vi "Make Project Title string.vi"(6 "Version":string, 8 "Simulate?":bool, 9 "Debug?":bool, 10 "Project Name":string) -> (3 "Title Bar":string)   [LabVIEW 2013, in "Strings Lib.lvlib"]
doc: "Formats the title bar string."
uses:
  Strings Lib.lvlib
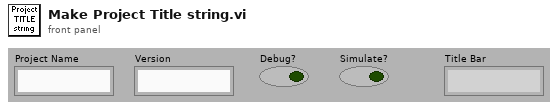
[diagram p1: front panel]
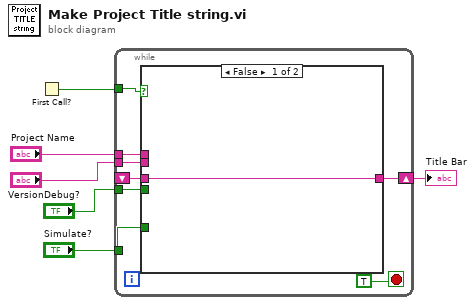
[diagram p0: block diagram]
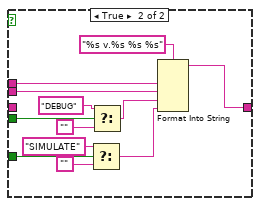
[diagram p2: hidden frame]
diagram:
  n1 = First Call?() -> (First Call?: T/F=w1:bool)
  n2 = while {
    tunnel: "Simulate?" -> [w13]
    tunnel: "Debug?" -> [w12]
    tunnel: "Version" -> [w11]
    tunnel: "Project Name" -> [w10]
    tunnel: w1 -> [w9]
    shift-right: [w14] -> w6
    shift-left: _ -> [w8]
    stop <- TRUE stop-if-true
    n3 = case shown="False" w9 {
      tunnel: [w15 w22] -> w14
      tunnel: w13 -> [_ w20]
      tunnel: w12 -> [_ w19]
      tunnel: w11 -> [_ w18]
      tunnel: w10 -> [_ w16]
      tunnel: w8 -> [w15 _]
      frame False {
      }
      frame True {
        n4 = Select(t="SIMULATE" ("format string"), s=w20, f="") -> (s? t:f=w26:string)
        n5 = Select(t="DEBUG" ("format string"), s=w19, f="") -> (s? t:f=w27:string)
        n6 = Format Into String(format string="%s v.%s %s %s", w16, w18, w27, w26) -> (resulting string=w22:string)  [unwired: 2 in, 1 out]
      }
    }
  }
  "Title Bar" <- w6
